vi "Read File and Calculate.vi"(11 "file path (dialog if empty)":path) -> (3 "Cluster":T1)   [LabVIEW 2019, in "SME_Report.lvlib"]
uses:
  <vilib>/Utility/file.llb/Read Delimited Spreadsheet (string).vi
  SME_Report.lvlib
  <vilib>/Analysis/NI_AALBase.lvlib
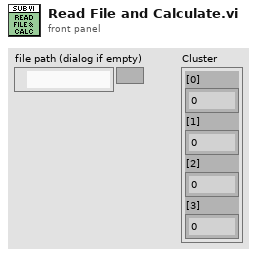
[diagram p1: front panel]
types:
  T1 = cluster{"[0]":dbl, "[1]":dbl, "[2]":dbl, "[3]":dbl}
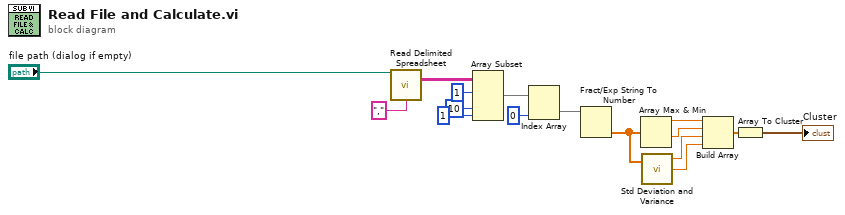
[diagram p0: block diagram]
diagram:
  n1 = call-poly <vilib>:"Read Delimited Spreadsheet.vi"("file path (dialog if empty)"="file path (dialog if empty)", "delimiter (\\t)"="," ("delimiter (\\t)")) -> ("all rows"=w2:string[][])  [unwired: 8 in, 5 out]
  n2 = Array Subset(array=w2, index (row)=1 ("index"), index (col)=10 ("index"), length (col)=1 ("length")) -> (w6:string[][])  [unwired: 1 in]
  n3 = Index Array(array=w6, index (col)=0 ("disabled index (col)")) -> (element=w8:string[])  [unwired: 1 in]
  n4 = Fract/Exp String To Number(string=w8) -> (number=w9:dbl[])  [unwired: 3 in, 1 out]
  n5 = Array Max & Min(array=w9) -> (max value=w10:dbl, min value=w11:dbl)  [unwired: 2 out]
  n6 = call <vilib>:"Std Deviation and Variance.vi"("X"=w9) -> ("mean"=w14:dbl, "standard deviation"=w13:dbl)  [unwired: 1 in, 1 out]
  n7 = Build Array(w10, w11, w14, w13) -> (w15:dbl[])
  n8 = Array To Cluster(array=w15) -> (cluster=→"Cluster":T1)
